vi "Calculate Current or Voltage Values, Source Delays and Time to Acquire.vi"(0 "Current/voltage start point (AorV)":dbl, 5 "Current/voltage end point (AorV)":dbl=3.0, 7 "Current/voltage slew rate (AorV/sec)":dbl=1000.0, 9 "Update Rate (S/sec)":dbl=1000.0, 11 "error in (no error)":errorcluster) -> (4 "Current or voltage values":dbl[](array[numeric]), 6 "Source delays (sec)":dbl[](array[numeric]), 8 "Time to acquire (sec)":dbl, 10 "Number of samples":i32, 15 "error out":errorcluster)   [LabVIEW 2021]
uses:
  <vilib>/Analysis/1siggen.llb/Ramp Pattern by Samples.vi
  <vilib>/Analysis/NI_AALBase.lvlib
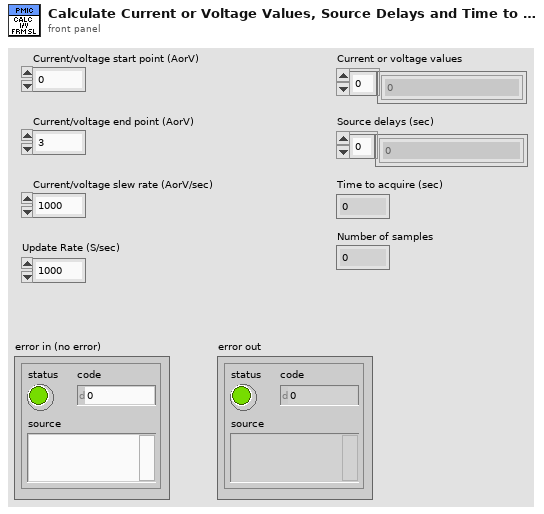
[diagram p1: front panel]
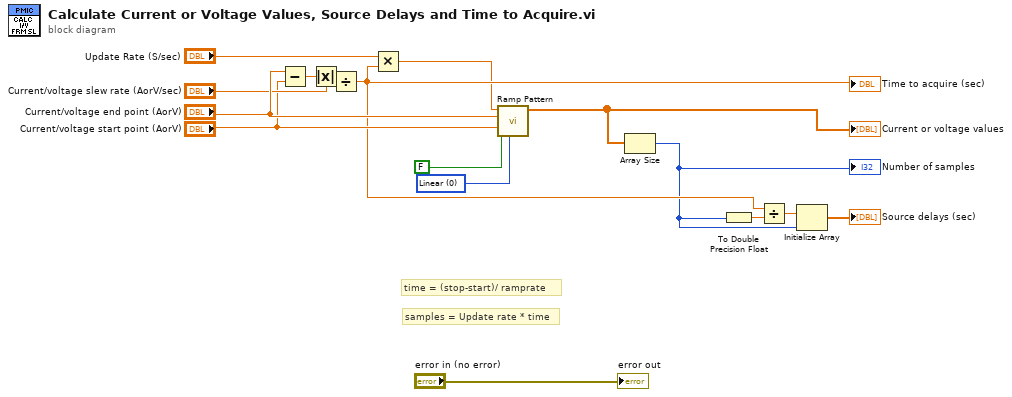
[diagram p0: block diagram]
diagram:
  w15 = u16 0 items=["Linear", "Logarithmic"] ("type")
  # "samples = Update rate * time"
  # "time = (stop-start)/ ramprate"
  n1 = Subtract(x="Current/voltage end point (AorV)", y="Current/voltage start point (AorV)") -> (x-y=w13:dbl)
  n2 = Absolute Value(x=w13) -> (abs(x)=w1:dbl)
  n3 = Divide(x=w1, y="Current/voltage slew rate (AorV/sec)") -> (x/y=w6:dbl)
  "Time to acquire (sec)" <- w6
  n4 = Multiply(x="Update Rate (S/sec)", y=w6) -> (x*y=w5:dbl)
  n5 = call-poly <vilib>:"Ramp Pattern.vi"("type"=w15, "exclude end?"=FALSE, "start"="Current/voltage start point (AorV)", "end"="Current/voltage end point (AorV)", "samples"=w5) -> ("Ramp Pattern"=w8:dbl[])  [unwired: 5 in, 1 out]
  "Current or voltage values" <- w8
  n6 = Array Size(array=w8) -> (size(s)=w3:i32)
  "Number of samples" <- w3
  n7 = To Double Precision Float(number=w3) -> (double precision float=w4:dbl)
  n8 = Divide(x=w6, y=w4) -> (x/y=w10:dbl)
  n9 = Initialize Array(w10, w3) -> (→"Source delays (sec)":dbl[])
  "error out" <- "error in (no error)"
